vi "Column Visibility.vi"(8 "error in (no error)":errorcluster, 9 "Visibility":bool[](array[boolean]), 10 "Column Indexes":i32[](array[numeric]), 11 "DataGridView in":refnum<class "DataGridView.lvclass">) -> (0 "error out":errorcluster, 3 "DataGridView out":refnum<class "DataGridView.lvclass">)   [LabVIEW 2013, in "DataGrid.lvlib" / "DataGridView.lvclass"]
doc: "Sets the visibility of any columns making it easy to how/hide column or groups of columns"
uses:
  DataGridView.lvclass
  System.Windows.Forms
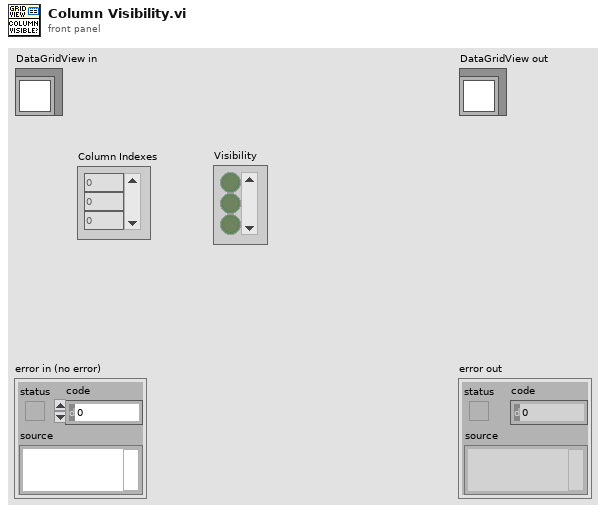
[diagram p1: front panel]
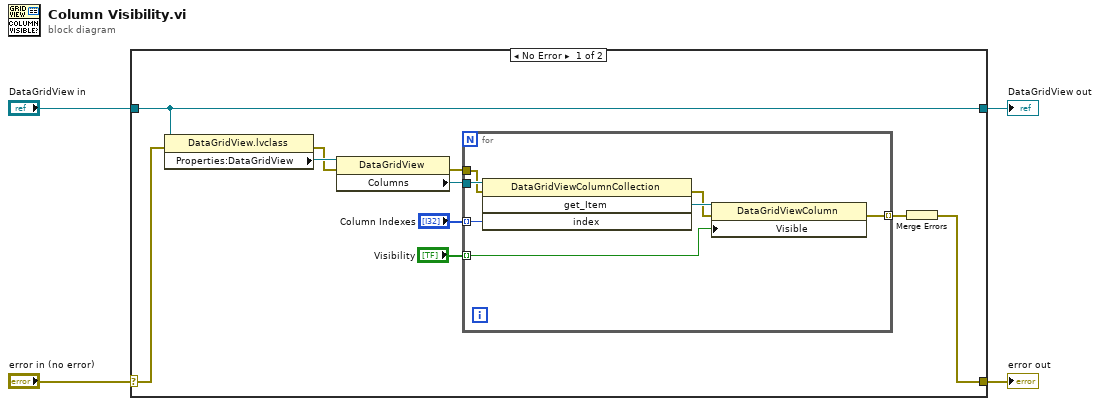
[diagram p0: block diagram]
diagram:
  n1 = case shown="No Error" "error in (no error)" {
    selector: "error in (no error)" -> [w12 w23]
    tunnel: [w5 w23] -> w3
    tunnel: [w14 w22] -> w1
    tunnel: "DataGridView in" -> [w14 w22]
    frame No Error {
      n2 = property class="DataGridView.lvclass"(reference=w14, error in=w12) -> (error out=w11:errorcluster, "Properties:DataGridView"=w13:refnum<k24>)  [unwired: 1 out]
      n3 = property class="DataGridView"(reference=w13, error in=w11) -> (error out=w7:errorcluster, "Columns"=w9:refnum<k24>)  [unwired: 1 out]
      n4 = for {
        tunnel: "Column Indexes" -> [w20] mode=indexing
        tunnel: w9 -> [w21]
        tunnel: "Visibility" -> [w18] mode=indexing
        tunnel: w7 -> [w17]
        tunnel: [w15] -> w6 mode=indexing
        n5 = invoke class="DataGridViewColumnCollection" method="get_Item"(reference=w21, error in=w17, "index"=w20) -> (error out=w16:errorcluster, "get_Item"=w19:refnum<k24>)  [unwired: 1 in, 2 out]
        n6 = property class="DataGridViewColumn"(reference=w19, error in=w16, "Visible"=w18) -> (error out=w15:errorcluster)  [unwired: 1 out]
      }
      n7 = Merge Errors(w6) -> (w5:errorcluster)
    }
    frame Error {
    }
  }
  "error out" <- w3
  "DataGridView out" <- w1
